vi "Test Deserialize Variant Attributes.vi"(8 "error in (no error)":errorcluster) -> (0 "error out":errorcluster)   [LabVIEW 2015]
uses:
  src/Deserializer/JSON Deserializer/JSON Deserializer.lvclass
  <vilib>/addons/_JKI Toolkits/Caraya/classes/Test/Test.lvclass
  <vilib>/addons/_JKI Toolkits/Caraya/classes/Assert/Assert.lvclass
  src/JKI JSON Serialization.lvlib
  <vilib>/Utility/Data Type/NI_Data Type.lvlib
panel:
  out "data 2":string
  out "value":variant
  in  "Google reverse-geocode results":string="{\n   \"results\" : [\n      {\n         \"address_components\" : [\n            {\n               \"long_name\" : \"The White House\",\n               \"short_name\" : \"The White House\",\n               \"types\" : [ \"premise\" ]\n            },\n            {\n               \"long_name\" : \"1600\",\n               \"short_name\" : \"1600\",\n               \"types\" : [ \"street_number\" ]\n            },\n            {\n               \"long_name\" : \"Pennsylvania Avenue Northwest\",\n               \"short_name\" : \"Pennsylvania Ave NW\",\n               \"types\" : [ \"route\" ]\n            },\n            {\n               \"long_name\" : \"Northwest Washington\",\n               \"short_name\" : \"Northwest Washington\",\n               \"types\" : [ \"neighborhood\", \"political\" ]\n            },\n            {\n               \"long_name\" : \"Washington\",\n               \"short_name\" : \"Washington\",\n               \"types\" : [ \"locality\", \"political\" ]\n            },\n            {\n               \"long_name\" : \"District of Columbia\",\n               \"short_name\" : \"DC\",\n               \"types\" : [ \"administrative_area_level_1\", \"political\" ]\n            },\n            {\n               \"long_name\" : \"United States\",\n               \"short_name\" : \"US\",\n               \"types\" : [ \"country\", \"political\" ]\n            },\n            {\n               \"long_name\" : \"20500\",\n               \"short_name\" : \"20500\",\n               \"types\" : [ \"postal_code\" ]\n            }\n         ],\n         \"formatted_address\" : \"The White House, 1600 Pennsylvania Ave NW, Washington, DC 20500, USA\",\n         \"geometry\" : {\n            \"bounds\" : {\n               \"northeast\" : {\n                  \"lat\" : 38.8979044,\n                  \"lng\" : -77.0355124\n               },\n               \"southwest\" : {\n                  \"lat\" : 38.8973144,\n                  \"lng\" : -77.03795749999999\n               }\n            },\n            \"location\" : {\n               \"lat\" : 38.8976094,\n               \"lng\" : -77.0367349\n            },\n            \"location_type\" : \"ROOFTOP\",\n            \"viewport\" : {\n               \"northeast\" : {\n                  \"lat\" : 38.8989583802915,\n                  \"lng\" : -77.03538596970849\n               },\n               \"southwest\" : {\n                  \"lat\" : 38.8962604197085,\n                  \"lng\" : -77.03808393029151\n               }\n            }\n         },\n         \"place_id\" : \"ChIJGVtI4by3t4kRr51d_Qm_x58\",\n         \"types\" : [ \"premise\" ]\n      },\n      {\n         \"address_components\" : [\n            {\n               \"long_name\" : \"West Executive Avenue Northwest\",\n               \"short_name\" : \"W Executive Ave NW\",\n               \"types\" : [ \"route\" ]\n            },\n            {\n               \"long_name\" : \"Northwest Washington\",\n               \"short_name\" : \"Northwest Washington\",\n               \"types\" : [ \"neighborhood\", \"political\" ]\n            },\n            {\n               \"long_name\" : \"Washington\",\n               \"short_name\" : \"Washington\",\n               \"types\" : [ \"locality\", \"political\" ]\n            },\n            {\n               \"long_name\" : \"District of Columbia\",\n               \"short_name\" : \"DC\",\n               \"types\" : [ \"administrative_area_level_1\", \"political\" ]\n            },\n            {\n               \"long_name\" : \"United States\",\n               \"short_name\" : \"US\",\n               \"types\" : [ \"country\", \"political\" ]\n            },\n            {\n               \"long_name\" : \"20500\",\n               \"short_name\" : \"20500\",\n               \"types\" : [ \"postal_code\" ]\n            }\n         ],\n         \"formatted_address\" : \"W Executive Ave NW, Washington, DC 20500, USA\",\n         \"geometry\" : {\n            \"bounds\" : {\n               \"northeast\" : {\n                  \"lat\" : 38.8987179,\n                  \"lng\" : -77.0379902\n               },\n               \"southwest\" : {\n                  \"lat\" : 38.8963906,\n                  \"lng\" : -77.0379916\n               }\n            },\n            \"location\" : {\n               \"lat\" : 38.89755419999999,\n               \"lng\" : -77.0379909\n            },\n            \"location_type\" : \"GEOMETRIC_CENTER\",\n            \"viewport\" : {\n               \"northeast\" : {\n                  \"lat\" : 38.8989032302915,\n                  \"lng\" : -77.03664191970849\n               },\n               \"southwest\" : {\n                  \"lat\" : 38.8962052697085,\n                  \"lng\" : -77.03933988029149\n               }\n            }\n         },\n         \"place_id\" : \"ChIJPWmSlby3t4kRBbzLK31n4RE\",\n         \"types\" : [ \"route\" ]\n      },\n      {\n         \"address_components\" : [\n            {\n               \"long_name\" : \"Northwest Washington\",\n               \"short_name\" : \"Northwest Washington\",\n               \"types\" : [ \"neighborhood\", \"political\" ]\n            },\n            {\n               \"long_name\" : \"Washington\",\n               \"short_name\" : \"Washington\",\n               \"types\" : [ \"locality\", \"political\" ]\n            },\n            {\n               \"long_name\" : \"District of Columbia\",\n               \"short_name\" : \"DC\",\n               \"types\" : [ \"administrative_area_level_1\", \"political\" ]\n            },\n            {\n               \"long_name\" : \"United States\",\n               \"short_name\" : \"US\",\n               \"types\" : [ \"country\", \"political\" ]\n            }\n         ],\n         \"formatted_address\" : \"Northwest Washington, Washington, DC, USA\",\n         \"geometry\" : {\n            \"bounds\" : {\n               \"northeast\" : {\n                  \"lat\" : 38.9955566,\n                  \"lng\" : -77.00605969999999\n               },\n               \"southwest\" : {\n                  \"lat\" : 38.8891955,\n                  \"lng\" : -77.1197502\n               }\n            },\n            \"location\" : {\n               \"lat\" : 38.9380912,\n               \"lng\" : -77.04493269999999\n            },\n            \"location_type\" : \"APPROXIMATE\",\n            \"viewport\" : {\n               \"northeast\" : {\n                  \"lat\" : 38.9955566,\n                  \"lng\" : -77.00605969999999\n               },\n               \"southwest\" : {\n                  \"lat\" : 38.8891955,\n                  \"lng\" : -77.1197502\n               }\n            }\n         },\n         \"place_id\" : \"ChIJi7U4CaS3t4kR0m_KoPJ00Bw\",\n         \"types\" : [ \"neighborhood\", \"political\" ]\n      },\n      {\n         \"address_components\" : [\n            {\n               \"long_name\" : \"Washington\",\n               \"short_name\" : \"Washington\",\n               \"types\" : [ \"locality\", \"political\" ]\n            },\n            {\n               \"long_name\" : \"District of Columbia\",\n               \"short_name\" : \"District of Columbia\",\n               \"types\" : [ \"administrative_area_level_2\", \"political\" ]\n            },\n            {\n               \"long_name\" : \"District of Columbia\",\n               \"short_name\" : \"DC\",\n               \"types\" : [ \"administrative_area_level_1\", \"political\" ]\n            },\n            {\n               \"long_name\" : \"United States\",\n               \"short_name\" : \"US\",\n               \"types\" : [ \"country\", \"political\" ]\n            }\n         ],\n         \"formatted_address\" : \"Washington, DC, USA\",\n         \"geometry\" : {\n            \"bounds\" : {\n               \"northeast\" : {\n                  \"lat\" : 38.995548,\n                  \"lng\" : -76.90939299999999\n               },\n               \"southwest\" : {\n                  \"lat\" : 38.8031494,\n                  \"lng\" : -77.1197401\n               }\n            },\n            \"location\" : {\n               \"lat\" : 38.9071923,\n               \"lng\" : -77.03687069999999\n            },\n            \"location_type\" : \"APPROXIMATE\",\n            \"viewport\" : {\n               \"northeast\" : {\n                  \"lat\" : 38.995548,\n                  \"lng\" : -76.90939299999999\n               },\n               \"southwest\" : {\n                  \"lat\" : 38.8031494,\n                  \"lng\" : -77.1197401\n               }\n            }\n         },\n         \"place_id\" : \"ChIJW-T2Wt7Gt4kRKl2I1CJFUsI\",\n         \"types\" : [ \"locality\", \"political\" ]\n      },\n      {\n         \"address_components\" : [\n            {\n               \"long_name\" : \"20502\",\n               \"short_name\" : \"20502\",\n               \"types\" : [ \"postal_code\" ]\n            },\n            {\n               \"long_name\" : \"Northwest Washington\",\n               \"short_name\" : \"Northwest Washington\",\n               \"types\" : [ \"neighborhood\", \"political\" ]\n            },\n            {\n               \"long_name\" : \"Washington\",\n               \"short_name\" : \"Washington\",\n               \"types\" : [ \"locality\", \"political\" ]\n            },\n            {\n               \"long_name\" : \"District of Columbia\",\n               \"short_name\" : \"DC\",\n               \"types\" : [ \"administrative_area_level_1\", \"political\" ]\n            },\n            {\n               \"long_name\" : \"United States\",\n               \"short_name\" : \"US\",\n               \"types\" : [ \"country\", \"political\" ]\n            }\n         ],\n         \"formatted_address\" : \"Washington, DC 20502, USA\",\n         \"geometry\" : {\n            \"bounds\" : {\n               \"northeast\" : {\n                  \"lat\" : 38.898761,\n                  \"lng\" : -77.03386789999999\n               },\n               \"southwest\" : {\n                  \"lat\" : 38.8926099,\n                  \"lng\" : -77.03848579999999\n               }\n            },\n            \"location\" : {\n               \"lat\" : 38.8967584,\n               \"lng\" : -77.03701629999999\n            },\n            \"location_type\" : \"APPROXIMATE\",\n            \"viewport\" : {\n               \"northeast\" : {\n                  \"lat\" : 38.898761,\n                  \"lng\" : -77.03386789999999\n               },\n               \"southwest\" : {\n                  \"lat\" : 38.8926099,\n                  \"lng\" : -77.03848579999999\n               }\n            }\n         },\n         \"place_id\" : \"ChIJFfZlI6O3t4kRT21JVHxrwx4\",\n         \"types\" : [ \"postal_code\" ]\n      },\n      {\n         \"address_components\" : [\n            {\n               \"long_name\" : \"20372\",\n               \"short_name\" : \"20372\",\n               \"types\" : [ \"postal_code\" ]\n            },\n            {\n               \"long_name\" : \"Washington\",\n               \"short_name\" : \"Washington\",\n               \"types\" : [ \"locality\", \"political\" ]\n            },\n            {\n               \"long_name\" : \"District of Columbia\",\n               \"short_name\" : \"DC\",\n               \"types\" : [ \"administrative_area_level_1\", \"political\" ]\n            },\n            {\n               \"long_name\" : \"United States\",\n               \"short_name\" : \"US\",\n               \"types\" : [ \"country\", \"political\" ]\n            }\n         ],\n         \"formatted_address\" : \"Washington, DC 20372, USA\",\n         \"geometry\" : {\n            \"bounds\" : {\n               \"northeast\" : {\n                  \"lat\" : 38.9103761,\n                  \"lng\" : -77.00899819999999\n               },\n               \"southwest\" : {\n                  \"lat\" : 38.8822807,\n                  \"lng\" : -77.0576224\n               }\n            },\n            \"location\" : {\n               \"lat\" : 38.8992416,\n               \"lng\" : -77.0303423\n            },\n            \"location_type\" : \"APPROXIMATE\",\n            \"viewport\" : {\n               \"northeast\" : {\n                  \"lat\" : 38.9103761,\n                  \"lng\" : -77.00899819999999\n               },\n               \"southwest\" : {\n                  \"lat\" : 38.8822807,\n                  \"lng\" : -77.0576224\n               }\n            }\n         },\n         \"place_id\" : \"ChIJGzCb9gq4t4kRN_0lpRhRhjU\",\n         \"types\" : [ \"postal_code\" ]\n      },\n      {\n         \"address_components\" : [\n            {\n               \"long_name\" : \"District of Columbia\",\n               \"short_name\" : \"DC\",\n               \"types\" : [ \"administrative_area_level_1\", \"political\" ]\n            },\n            {\n               \"long_name\" : \"United States\",\n               \"short_name\" : \"US\",\n               \"types\" : [ \"country\", \"political\" ]\n            }\n         ],\n         \"formatted_address\" : \"District of Columbia, USA\",\n         \"geometry\" : {\n            \"bounds\" : {\n               \"northeast\" : {\n                  \"lat\" : 38.995548,\n                  \"lng\" : -76.90939299999999\n               },\n               \"southwest\" : {\n                  \"lat\" : 38.8031494,\n                  \"lng\" : -77.1197401\n               }\n            },\n            \"location\" : {\n               \"lat\" : 38.9059849,\n               \"lng\" : -77.03341790000002\n            },\n            \"location_type\" : \"APPROXIMATE\",\n            \"viewport\" : {\n               \"northeast\" : {\n                  \"lat\" : 38.995548,\n                  \"lng\" : -76.90939299999999\n               },\n               \"southwest\" : {\n                  \"lat\" : 38.8031494,\n                  \"lng\" : -77.1197401\n               }\n            }\n         },\n         \"place_id\" : \"ChIJW-T2Wt7Gt4kRmKFUAsCO4tY\",\n         \"types\" : [ \"administrative_area_level_1\", \"political\" ]\n      },\n      {\n         \"address_components\" : [\n            {\n               \"long_name\" : \"Washington-Arlington-Alexandria, DC-VA-MD-WV\",\n               \"short_name\" : \"Washington-Arlington-Alexandria, DC-VA-MD-WV\",\n               \"types\" : [ \"political\" ]\n            },\n            {\n               \"long_name\" : \"United States\",\n               \"short_name\" : \"US\",\n               \"types\" : [ \"country\", \"political\" ]\n            }\n         ],\n         \"formatted_address\" : \"Washington-Arlington-Alexandria, DC-VA-MD-WV, USA\",\n         \"geometry\" : {\n            \"bounds\" : {\n               \"northeast\" : {\n                  \"lat\" : 39.720018,\n                  \"lng\" : -76.38622889999999\n               },\n               \"southwest\" : {\n                  \"lat\" : 37.9911599,\n                  \"lng\" : -78.38668199999999\n               }\n            },\n            \"location\" : {\n               \"lat\" : 39.1289725,\n               \"lng\" : -77.3783789\n            },\n            \"location_type\" : \"APPROXIMATE\",\n            \"viewport\" : {\n               \"northeast\" : {\n                  \"lat\" : 39.720023,\n                  \"lng\" : -76.38622889999999\n               },\n               \"southwest\" : {\n                  \"lat\" : 37.9911599,\n                  \"lng\" : -78.38668199999999\n               }\n            }\n         },\n         \"place_id\" : \"ChIJy25QE7lFtokRgaAnbc9iMr8\",\n         \"types\" : [ \"political\" ]\n      },\n      {\n         \"address_components\" : [\n            {\n               \"long_name\" : \"United States\",\n               \"short_name\" : \"US\",\n               \"types\" : [ \"country\", \"political\" ]\n            }\n         ],\n         \"formatted_address\" : \"United States\",\n         \"geometry\" : {\n            \"bounds\" : {\n               \"northeast\" : {\n                  \"lat\" : 71.3867745,\n                  \"lng\" : -66.9502861\n               },\n               \"southwest\" : {\n                  \"lat\" : 18.910677,\n                  \"lng\" : 172.4458955\n               }\n            },\n            \"location\" : {\n               \"lat\" : 37.09024,\n               \"lng\" : -95.712891\n            },\n            \"location_type\" : \"APPROXIMATE\",\n            \"viewport\" : {\n               \"northeast\" : {\n                  \"lat\" : 49.38,\n                  \"lng\" : -66.94\n               },\n               \"southwest\" : {\n                  \"lat\" : 25.82,\n                  \"lng\" : -124.39\n               }\n            }\n         },\n         \"place_id\" : \"ChIJCzYy5IS16lQRQrfeQ5K5Oxw\",\n         \"types\" : [ \"country\", \"political\" ]\n      }\n   ],\n   \"status\" : \"OK\"\n}\n"
  out "Void Variant with Data as Attributes":variant
  out "JSON String":string
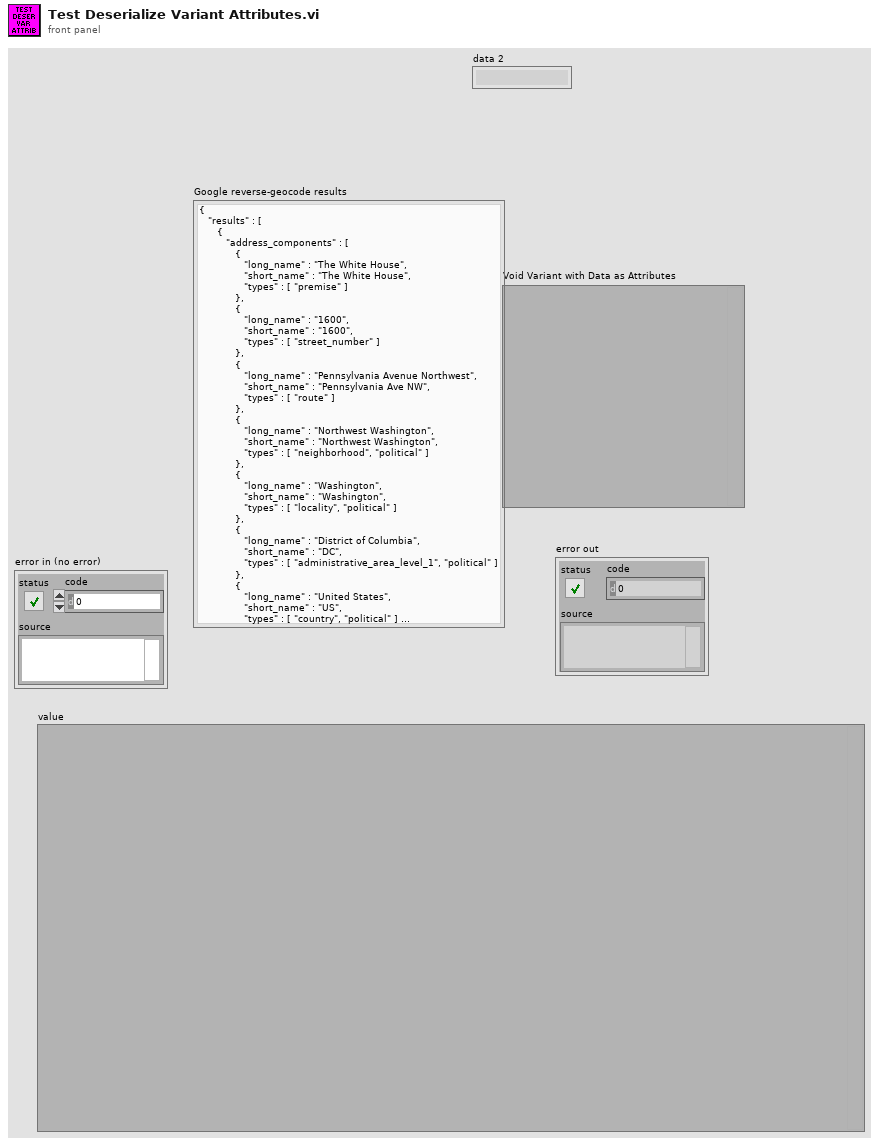
[diagram p1: front panel]
types:
  T1 = typedef "NI_Data Type.lvlib/Data Type.ctl" = enum8{"Invalid Type", "Void", "I8", "I16", "I32", "I64", "U8", "U16", "U32", "U64", "Single Float", "Double Float", "Extended Float", "Single Complex", "Double Complex", "Extended Complex", "Enum U8", "Enum U16", "Enum U32", "Enum U64", "Single Float With Unit", "Double Float With Unit", "Extended Float With Unit", "Single Complex with Unit", "Double Complex with Unit", "Extended Complex with Unit", "Boolean", "String", "Path", "Picture", "Tag", "Array", "Cluster", "Variant", "LV Variant", "Waveform", "Timestamp", "Digital Waveform", "Digital Data", "ExpressData", "Refnum", "External Data", "VI", "Poly VI", "LabVIEW Class Instance", "Fixed Point"}
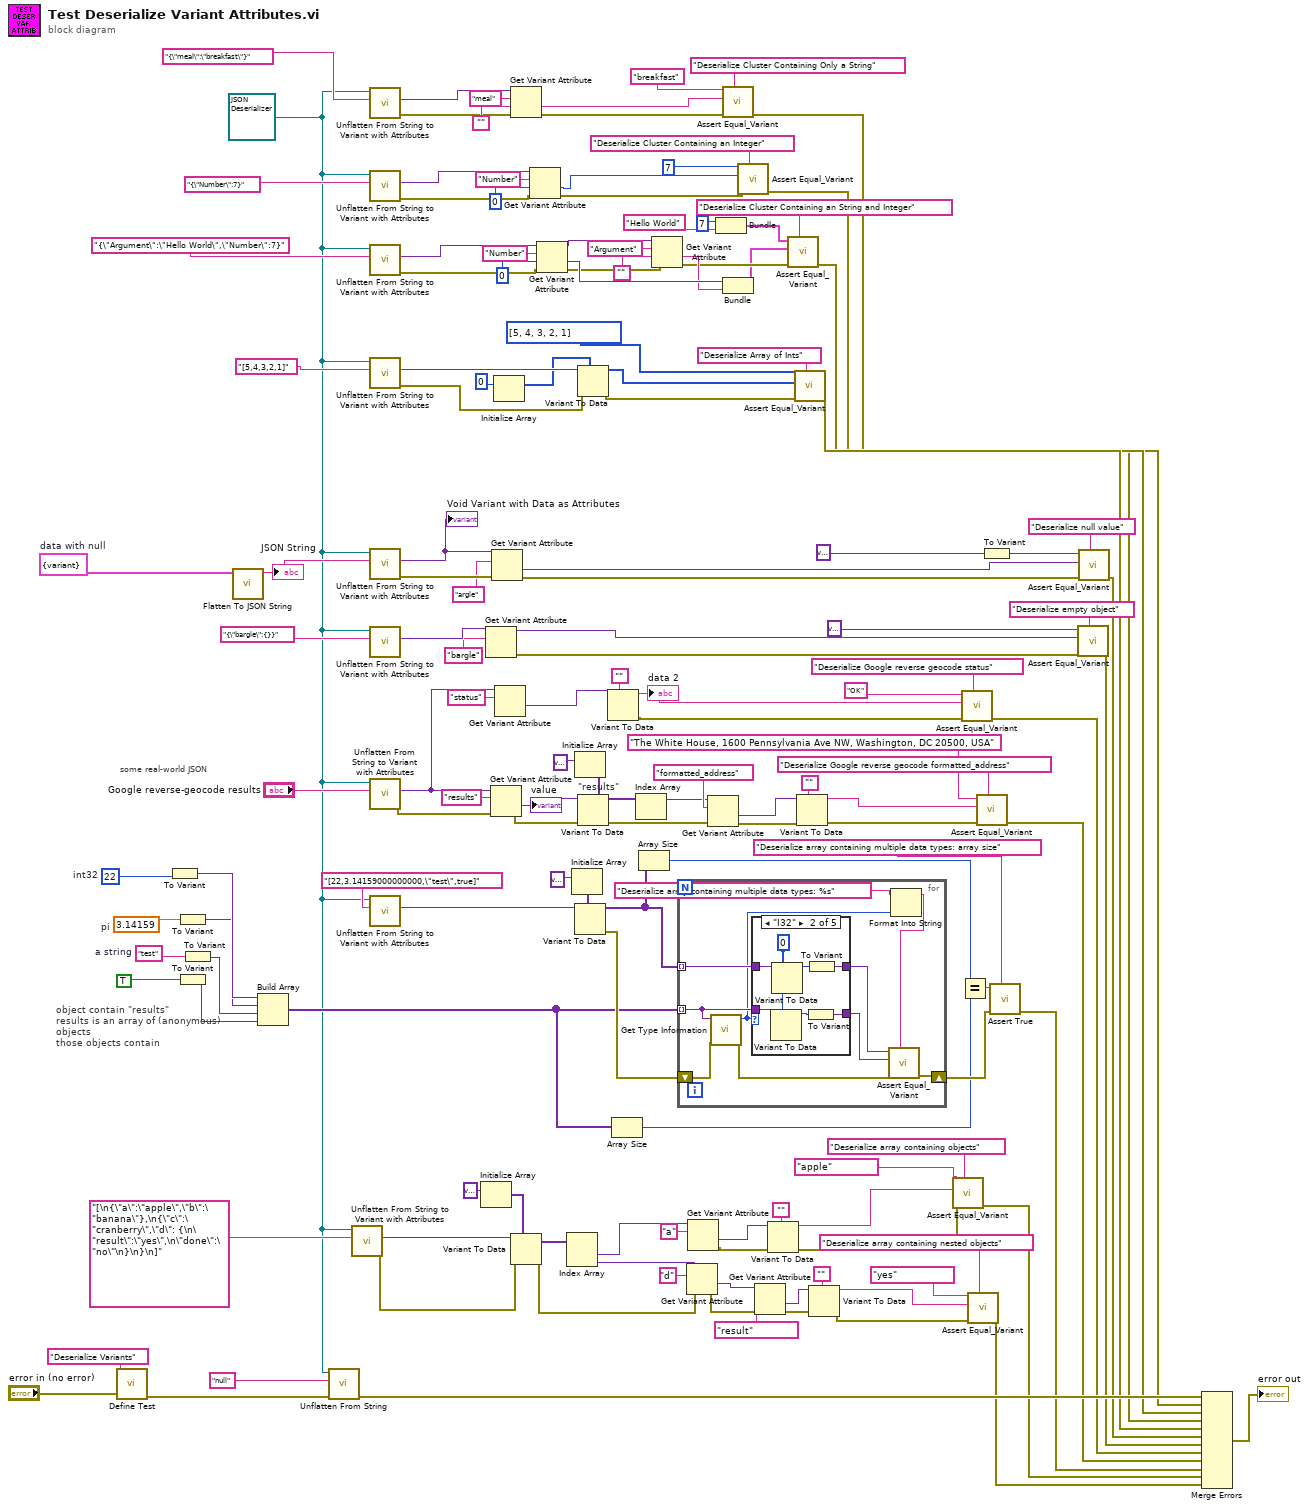
[diagram p0: block diagram]
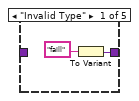
[diagram p2: hidden frame]
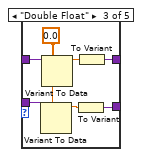
[diagram p3: hidden frame]
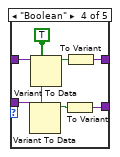
[diagram p4: hidden frame]
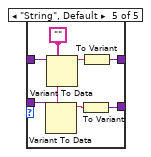
[diagram p5: hidden frame]
diagram:
  w22 = refnum<class "JSON Deserializer.lvclass"> refnum ("Deserializer out")
  w120 = "test"  # a string
  w116 = 3.14159  # pi
  w121 = 22  # int32
  w143 = cluster{"argle":variant} {"argle"=variant}  # data with null
  # "some real-world JSON"
  # "object contain \"results\"\nresults is an array of (anonymous) objects\nthose objects contain"
  n1 = call <vilib>:"Define Test.vi"("error in (no error)"="error in (no error)", "Label (VI Title)"="Deserialize Variants") -> ("error out"=w144:errorcluster)  [unwired: 9 in]
  n2 = To Variant(anything=w121) -> (Variant=w119:variant)
  n3 = To Variant(anything=w116) -> (Variant=w118:variant)
  n4 = To Variant(anything=TRUE) -> (Variant=w114:variant)
  n5 = To Variant(anything=w120) -> (Variant=w117:variant)
  n6 = call "Flatten To JSON String.vi"("Variant"=w143) -> ("JSON String"=w142:string)  [unwired: 9 in, 1 out]
  "JSON String" <- w142
  n7 = Build Array(w119, w118, w117, w114) -> (w33:variant[])
  n8 = call-dynamic "Unflatten From String.vi"("error in (no error)"=w144, "String"="null", "Deserializer in"=w22) -> ("error out"=w153:errorcluster)  [unwired: 6 in, 2 out]
  n9 = call-dynamic "Unflatten From String to Variant with Attributes.vi"("String"="[\n{\"a\":\"apple\",\"b\":\"banana\"},\n{\"c\":\"cranberry\",\"d\": {\n\"result\":\"yes\",\n\"done\":\"no\"\n}\n}\n]", "Deserializer in"=w22) -> ("error out"=w12:errorcluster, "Variant with Attributes"=w27:variant)  [unwired: 7 in, 1 out]
  n10 = call-dynamic "Unflatten From String to Variant with Attributes.vi"("String"="{\"meal\":\"breakfast\"}" ("String 2"), "Deserializer in"=w22) -> ("error out"=w82:errorcluster, "Variant with Attributes"=w84:variant)  [unwired: 7 in, 1 out]
  n11 = call-dynamic "Unflatten From String to Variant with Attributes.vi"("String"="{\"Number\":7}", "Deserializer in"=w22) -> ("error out"=w72:errorcluster, "Variant with Attributes"=w55:variant)  [unwired: 7 in, 1 out]
  n12 = call-dynamic "Unflatten From String to Variant with Attributes.vi"("String"="{\"Argument\":\"Hello World\",\"Number\":7}", "Deserializer in"=w22) -> ("error out"=w71:errorcluster, "Variant with Attributes"=w56:variant)  [unwired: 7 in, 1 out]
  n13 = call-dynamic "Unflatten From String to Variant with Attributes.vi"("String"="[5,4,3,2,1]", "Deserializer in"=w22) -> ("error out"=w91:errorcluster, "Variant with Attributes"=w96:variant)  [unwired: 7 in, 1 out]
  n14 = call-dynamic "Unflatten From String to Variant with Attributes.vi"("String"=w142, "Deserializer in"=w22) -> ("error out"=w141:errorcluster, "Variant with Attributes"=w140:variant)  [unwired: 7 in, 1 out]
  "Void Variant with Data as Attributes" <- w140
  n15 = call-dynamic "Unflatten From String to Variant with Attributes.vi"("String"="{\"bargle\":{}}" ("JSON String 2"), "Deserializer in"=w22) -> ("Variant with Attributes"=w131:variant)  [unwired: 7 in, 2 out]
  n16 = call-dynamic "Unflatten From String to Variant with Attributes.vi"("String"="Google reverse-geocode results", "Deserializer in"=w22) -> ("error out"=w47:errorcluster, "Variant with Attributes"=w103:variant)  [unwired: 7 in, 1 out]
  n17 = call-dynamic "Unflatten From String to Variant with Attributes.vi"("String"="[22,3.14159000000000,\"test\",true]", "Deserializer in"=w22) -> ("Variant with Attributes"=w111:variant)  [unwired: 7 in, 2 out]
  n18 = Initialize Array(variant) -> (w25:variant[])  [unwired: 1 in]
  n19 = Get Variant Attribute(Variant=w131, name="bargle") -> (duplicate Variant=w127:variant, error out=w54:errorcluster)  [unwired: 2 in, 2 out]
  n20 = Get Variant Attribute(Variant=w103, name="results", error in=w47) -> (value=w107:variant, error out=w46:errorcluster)  [unwired: 1 in, 2 out]
  "value" <- w107
  n21 = Get Variant Attribute(Variant=w140, name="argle", error in=w141) -> (value=w137:variant, error out=w138:errorcluster)  [unwired: 1 in, 2 out]
  n22 = Initialize Array(0) -> (w93:i32[])  [unwired: 1 in]
  n23 = Get Variant Attribute(Variant=w103, name="status") -> (value=w101:variant)  [unwired: 2 in, 3 out]
  n24 = Get Variant Attribute(Variant=w84, name="meal", default value (empty Variant)="", error in=w82) -> (value=w80:string, error out=w81:errorcluster)  [unwired: 2 out]
  n25 = Variant To Data(error in=w12, type=w25, Variant=w27) -> (data=w24:variant[], error out=w13:errorcluster)
  n26 = Get Variant Attribute(Variant=w55, name="Number", default value (empty Variant)=0, error in=w72) -> (value=w74:i32, error out=w73:errorcluster)  [unwired: 2 out]
  n27 = Get Variant Attribute(Variant=w56, name="Number", default value (empty Variant)=0, error in=w71) -> (duplicate Variant=w66:variant, value=w64:i32, error out=w60:errorcluster)  [unwired: 1 out]
  n28 = Index Array(array=w24) -> (element #1=w10:variant, element #2=w28:variant)  [unwired: 2 in]
  n29 = Initialize Array(variant) -> (w112:variant[])  [unwired: 1 in]
  n30 = Initialize Array(variant) -> (w108:variant[])  [unwired: 1 in]
  n31 = Variant To Data(type=w112, Variant=w111) -> (data=w37:variant[], error out=w35:errorcluster)  [unwired: 1 in]
  n32 = Variant To Data(error in=w91, type=w93, Variant=w96) -> (data=w92:i32[], error out=w90:errorcluster)
  n33 = Variant To Data "\"results\""(error in=w46, type=w108, Variant=w107) -> (data=w106:variant[], error out=w45:errorcluster)
  n34 = Variant To Data(type="", Variant=w101) -> (data=w52:string, error out=w53:errorcluster)  [unwired: 1 in]
  "data 2" <- w52
  n35 = Array Size(array=w33) -> (size(s)=w32:i32)
  n36 = Index Array(array=w106) -> (element=w99:variant)  [unwired: 1 in]
  n37 = Array Size(array=w37) -> (size(s)=w36:i32)
  n38 = Get Variant Attribute(Variant=w66, name="Argument", default value (empty Variant)="", error in=w60) -> (value=w63:string, error out=w59:errorcluster)  [unwired: 2 out]
  n39 = for {
    tunnel: w33 -> [w162] mode=indexing
    tunnel: w37 -> [w163] mode=indexing
    shift-right: [w159] -> w34
    shift-left: w35 -> [w161]
    n40 = call <vilib>:"Get Type Information.vi"("error in (no error)"=w161, "Variant"=w162) -> ("error out"=w160:errorcluster, "Type"=w155:T1)  [unwired: 5 in, 3 out]
    n41 = case shown="\"I32\"" w155 {
      tunnel: w163 -> [_ w172 w179 w186 w193]
      tunnel: w162 -> [_ w171 w178 w185 w192]
      tunnel: [w164 w169 w176 w183 w190] -> w158
      tunnel: [_ w167 w174 w181 w188] -> w157
      frame "Invalid Type" {
        n42 = To Variant(anything="faill" ("name")) -> (Variant=w164:variant)
      }
      frame "I32" {
        w166 = 0
        n43 = Variant To Data(type=w166, Variant=w171) -> (data=w168:i32)  [unwired: 1 in, 1 out]
        n44 = Variant To Data(type=w166, Variant=w172) -> (data=w170:i32)  [unwired: 1 in, 1 out]
        n45 = To Variant(anything=w168) -> (Variant=w167:variant)
        n46 = To Variant(anything=w170) -> (Variant=w169:variant)
      }
      frame "Double Float" {
        w173 = 0.0
        n47 = Variant To Data(type=w173, Variant=w178) -> (data=w175:dbl)  [unwired: 1 in, 1 out]
        n48 = Variant To Data(type=w173, Variant=w179) -> (data=w177:dbl)  [unwired: 1 in, 1 out]
        n49 = To Variant(anything=w175) -> (Variant=w174:variant)
        n50 = To Variant(anything=w177) -> (Variant=w176:variant)
      }
      frame "Boolean" {
        w180 = TRUE
        n51 = Variant To Data(type=w180, Variant=w185) -> (data=w182:bool)  [unwired: 1 in, 1 out]
        n52 = Variant To Data(type=w180, Variant=w186) -> (data=w184:bool)  [unwired: 1 in, 1 out]
        n53 = To Variant(anything=w182) -> (Variant=w181:variant)
        n54 = To Variant(anything=w184) -> (Variant=w183:variant)
      }
      frame "String", Default {
        w187 = ""
        n55 = Variant To Data(type=w187, Variant=w192) -> (data=w189:string)  [unwired: 1 in, 1 out]
        n56 = Variant To Data(type=w187, Variant=w193) -> (data=w191:string)  [unwired: 1 in, 1 out]
        n57 = To Variant(anything=w189) -> (Variant=w188:variant)
        n58 = To Variant(anything=w191) -> (Variant=w190:variant)
      }
    }
    n59 = Format Into String(format string="Deserialize array containing multiple data types: %s" ("Label"), w155) -> (resulting string=w154:string)  [unwired: 2 in, 1 out]
    n60 = call <vilib>:"Assert Equal_Variant.vi"("Label"=w154, "error in (no error)"=w160, "Y"=w157, "X"=w158) -> ("error out"=w159:errorcluster)  [unwired: 7 in]
  }
  n61 = Get Variant Attribute(Variant=w28, name="d", error in=w13) -> (value=w30:variant, error out=w14:errorcluster)  [unwired: 1 in, 2 out]
  n62 = Get Variant Attribute(Variant=w10, name="a") -> (value=w7:variant, error out=w8:errorcluster)  [unwired: 2 in, 2 out]
  n63 = Get Variant Attribute(Variant=w99, name="formatted_address", error in=w45) -> (value=w100:variant, error out=w44:errorcluster)  [unwired: 1 in, 2 out]
  n64 = Bundle(7, "name"="Hello World") -> (w58:cluster{i32, "name":string})  [unwired: 1 in]
  n65 = call <vilib>:"Assert Equal_Variant.vi"("Label"="Deserialize Cluster Containing Only a String", "error in (no error)"=w81, "Y"=w80, "X"="breakfast" ("name")) -> ("error out"=w146:errorcluster)  [unwired: 7 in]
  n66 = Bundle(w64, w63) -> (w57:cluster{i32, string})  [unwired: 1 in]
  n67 = call <vilib>:"Assert Equal_Variant.vi"("Label"="Deserialize Cluster Containing an Integer", "error in (no error)"=w73, "Y"=w74, "X"=7) -> ("error out"=w147:errorcluster)  [unwired: 7 in]
  n68 = Get Variant Attribute(Variant=w30, name="result", error in=w14) -> (value=w19:variant, error out=w20:errorcluster)  [unwired: 1 in, 2 out]
  n69 = Variant To Data(error in=w8, type="", Variant=w7) -> (data=w5:string, error out=w4:errorcluster)
  n70 = call <vilib>:"Assert Equal_Variant.vi"("Label"="Deserialize Cluster Containing an String and Integer", "error in (no error)"=w59, "Y"=w57, "X"=w58) -> ("error out"=w145:errorcluster)  [unwired: 7 in]
  n71 = call <vilib>:"Assert Equal_Variant.vi"("Label"="Deserialize Array of Ints", "error in (no error)"=w90, "Y"=w92, "X"=i32[] [5, 4, 3, 2, 1]) -> ("error out"=w150:errorcluster)  [unwired: 7 in]
  n72 = Variant To Data(error in=w44, type="", Variant=w100) -> (data=w49:string, error out=w43:errorcluster)
  n73 = Variant To Data(error in=w20, type="", Variant=w19) -> (data=w17:string, error out=w15:errorcluster)
  n74 = call <vilib>:"Assert Equal_Variant.vi"("Label"="Deserialize array containing objects", "error in (no error)"=w4, "Y"=w5, "X"="apple" ("name")) -> ("error out"=w2:errorcluster)  [unwired: 7 in]
  n75 = Equal?(x=w36, y=w32) -> (x = y?=w110:bool)
  n76 = call <vilib>:"Assert Equal_Variant.vi"("Label"="Deserialize Google reverse geocode status", "error in (no error)"=w53, "Y"=w52, "X"="OK" ("data 3")) -> ("error out"=w48:errorcluster)  [unwired: 7 in]
  n77 = call <vilib>:"Assert Equal_Variant.vi"("Label"="Deserialize array containing nested objects", "error in (no error)"=w15, "Y"=w17, "X"="yes" ("name")) -> ("error out"=w3:errorcluster)  [unwired: 7 in]
  n78 = call <vilib>:"Assert Equal_Variant.vi"("Label"="Deserialize Google reverse geocode formatted_address", "error in (no error)"=w43, "Y"=w49, "X"="The White House, 1600 Pennsylvania Ave NW, Washington, DC 20500, USA" ("data 3")) -> ("error out"=w42:errorcluster)  [unwired: 7 in]
  n79 = To Variant(anything=variant) -> (Variant=w133:variant)
  n80 = call <vilib>:"Assert True.vi"("Label"="Deserialize array containing multiple data types: array size", "error in (no error)"=w34, "True?"=w110) -> ("error out"=w40:errorcluster)  [unwired: 8 in]
  n81 = call <vilib>:"Assert Equal_Variant.vi"("Label"="Deserialize empty object", "error in (no error)"=w54, "Y"=w127, "X"=variant) -> ("error out"=w126:errorcluster)  [unwired: 7 in]
  n82 = call <vilib>:"Assert Equal_Variant.vi"("Label"="Deserialize null value", "error in (no error)"=w138, "Y"=w137, "X"=w133) -> ("error out"=w135:errorcluster)  [unwired: 7 in]
  n83 = Merge Errors(w153, w146, w147, w145, w150, w135, w126, w48, w42, w40, w2, w3) -> (→"error out":errorcluster)
